vi "Speech-SpeakText.vi"(8 "error in (no error)":errorcluster, 10 "text to be spoken":string, 11 "speech_voice_refs (in)":T1) -> (0 "error out":errorcluster, 3 "speech_voice_refs (out)":T1)   [LabVIEW 8.6]
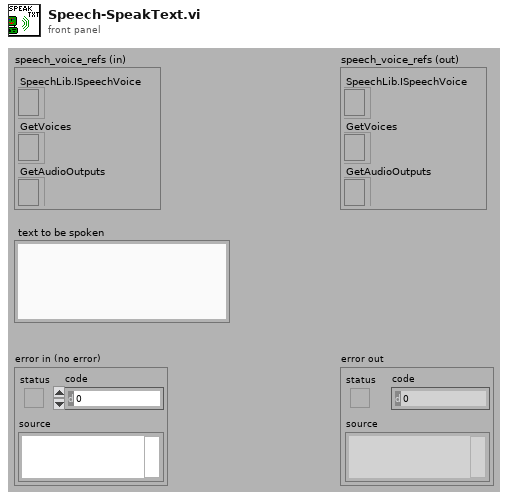
[diagram p1: front panel]
types:
  T1 = cluster{"SpeechLib.ISpeechVoice":refnum<k7>, "GetVoices":refnum<k7>, "GetAudioOutputs":refnum<k7>}
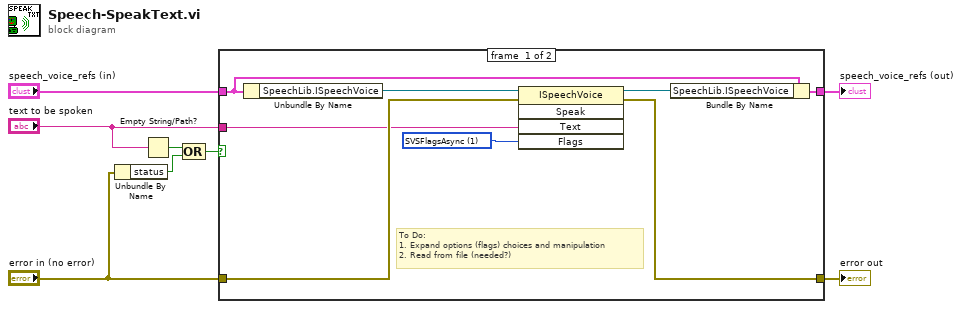
[diagram p0: block diagram]
diagram:
  n1 = Unbundle By Name("error in (no error)") -> ("status"=w3:bool)
  n2 = Empty String/Path?(string/path="text to be spoken") -> (empty?=w4:bool)
  n3 = Compound Arithmetic op=OR(w4, w3) -> (w2:bool)
  n4 = case shown="False" w2 {
    tunnel: "speech_voice_refs (in)" -> [w16 w17]
    tunnel: [w15 w18] -> w7
    tunnel: [w14 w17] -> w6
    tunnel: "error in (no error)" -> [w13 w18]
    tunnel: "text to be spoken" -> [w12 _]
    frame #0 {
      w9 = 1 items=["SVSFDefault", "SVSFlagsAsync", "SVSFPurgeBeforeSpeak", "SVSFIsFilename", "SVSFIsXML", "SVSFIsNotXML", "SVSFPersistXML", "SVSFNLPSpeakPunc, SVSFNLPMask", "SVSFVoiceMask", "SVSFUnusedFlags"] ("Flags")
      # "To Do:\n1. Expand options (flags) choices and manipulation\n2. Read from file (needed?)"
      n5 = Unbundle By Name(w16) -> ("SpeechLib.ISpeechVoice"=w11:refnum<k7>)
      n6 = invoke class="ISpeechVoice" method="Speak"(reference=w11, error in=w13, "Text"=w12, "Flags"=w9) -> (reference out=w10:refnum<k7>, error out=w15:errorcluster)  [unwired: 1 in, 3 out]
      n7 = Bundle By Name(cluster=w16, "SpeechLib.ISpeechVoice"=w10) -> (w14:T1)
    }
    frame #1 {
    }
  }
  "error out" <- w7
  "speech_voice_refs (out)" <- w6
